vi "Get Module Name.vi"(8 "error in (no error)":errorcluster, 9 "slot number":u32, 10 "chassis":refnum<k21>, 11 "session in":refnum<k21>) -> (0 "error out":errorcluster, 1 "module present?":bool, 2 "module":refnum<k21>, 3 "session out":refnum<k21>)   [LabVIEW 2020, in "SLSC.lvlib"]
doc: "Gets the name of a module on the chassis."
uses:
  <vilib>/SLSC/SLSC.lvlib
  <resource>/objmgr/slsc.rc
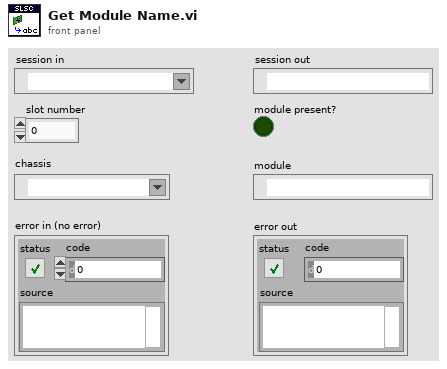
[diagram p1: front panel]
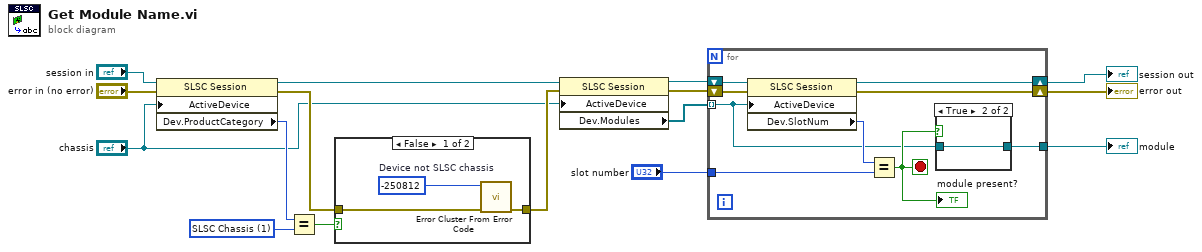
[diagram p0: block diagram]
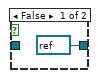
[diagram p3: hidden frame]
diagram:
  w7 = 1 items=["Unknown", "SLSC Chassis", "SLSC Module"] ("Dev.ProductCategory")
  n1 = property class="SLSC Session"(reference="session in", error in="error in (no error)", "ActiveDevice"="chassis") -> (reference out=w6:refnum<k21>, error out=w9:errorcluster, "Dev.ProductCategory"=w8:i32)
  n2 = Equal?(x=w8, y=w7) -> (x = y?=w10:bool)
  n3 = case shown="False" w10 {
    tunnel: w9 -> [w19 w20]
    tunnel: [w17 w20] -> w5
    frame False {
      w18 = -250812  # Device not SLSC chassis
      n4 = call <vilib>:"Error Cluster From Error Code.vi"("error in (no error)"=w19, "error code (0)"=w18) -> ("error out"=w17:errorcluster)  [unwired: 7 in]
    }
    frame True {
    }
  }
  n5 = property class="SLSC Session"(reference=w6, error in=w5, "ActiveDevice"="chassis") -> (reference out=w3:refnum<k21>, error out=w4:errorcluster, "Dev.Modules"=w1:refnum<k21>[])
  n6 = for {
    shift-right: [w27] -> w12
    shift-left: w3 -> [w29]
    shift-right: [w26] -> w11
    shift-left: w4 -> [w28]
    tunnel: w1 -> [w21] mode=indexing
    tunnel: "slot number" -> [w25]
    tunnel: [w23] -> w15
    stop <- w24 stop-if-true
    n7 = property class="SLSC Session"(reference=w29, error in=w28, "ActiveDevice"=w21) -> (reference out=w27:refnum<k21>, error out=w26:errorcluster, "Dev.SlotNum"=w22:u32)
    n8 = Equal?(x=w22, y=w25) -> (x = y?=w24:bool)
    "module present?" <- w24
    n9 = case shown="True" w24 {
      tunnel: w21 -> [_ w31]
      tunnel: [refnum<k21> refnum ("SLSC Device") w31] -> w23
      frame False {
      }
      frame True {
      }
    }
  }
  "module" <- w15
  "session out" <- w12
  "error out" <- w11
